vi "SwerveDriveRotate.vi"(0 "Strafe Joystick Axes":cluster{"X":dbl, "Y":dbl}, 1 "Center of Rotation Joystick Axes":cluster{"X":dbl, "Y":dbl}, 3 "Trigger Axes":cluster{"Left":dbl, "Right":dbl}, 4 "Angle (degrees; 0 = right)":dbl, 5 "error in (no error)":errorcluster, 6 "Strafe Multiplier":dbl, 7 "FieldCentric? (T)":bool=TRUE, 8 "Rotation Multiplier":dbl, 10 "Max Wheel Speed":dbl) -> (19 "error out":errorcluster)   [LabVIEW 2014]
uses:
  Robot Global Data.vi
panel:
  in  "Motor Controller":T1(ring)
  out "Waveform Chart":cluster{"FL Speed":dbl, "Encoder Velocity":dbl}(graph)
  in  "set":bool
  in  "D":dbl
  in  "I":dbl
  in  "P":dbl
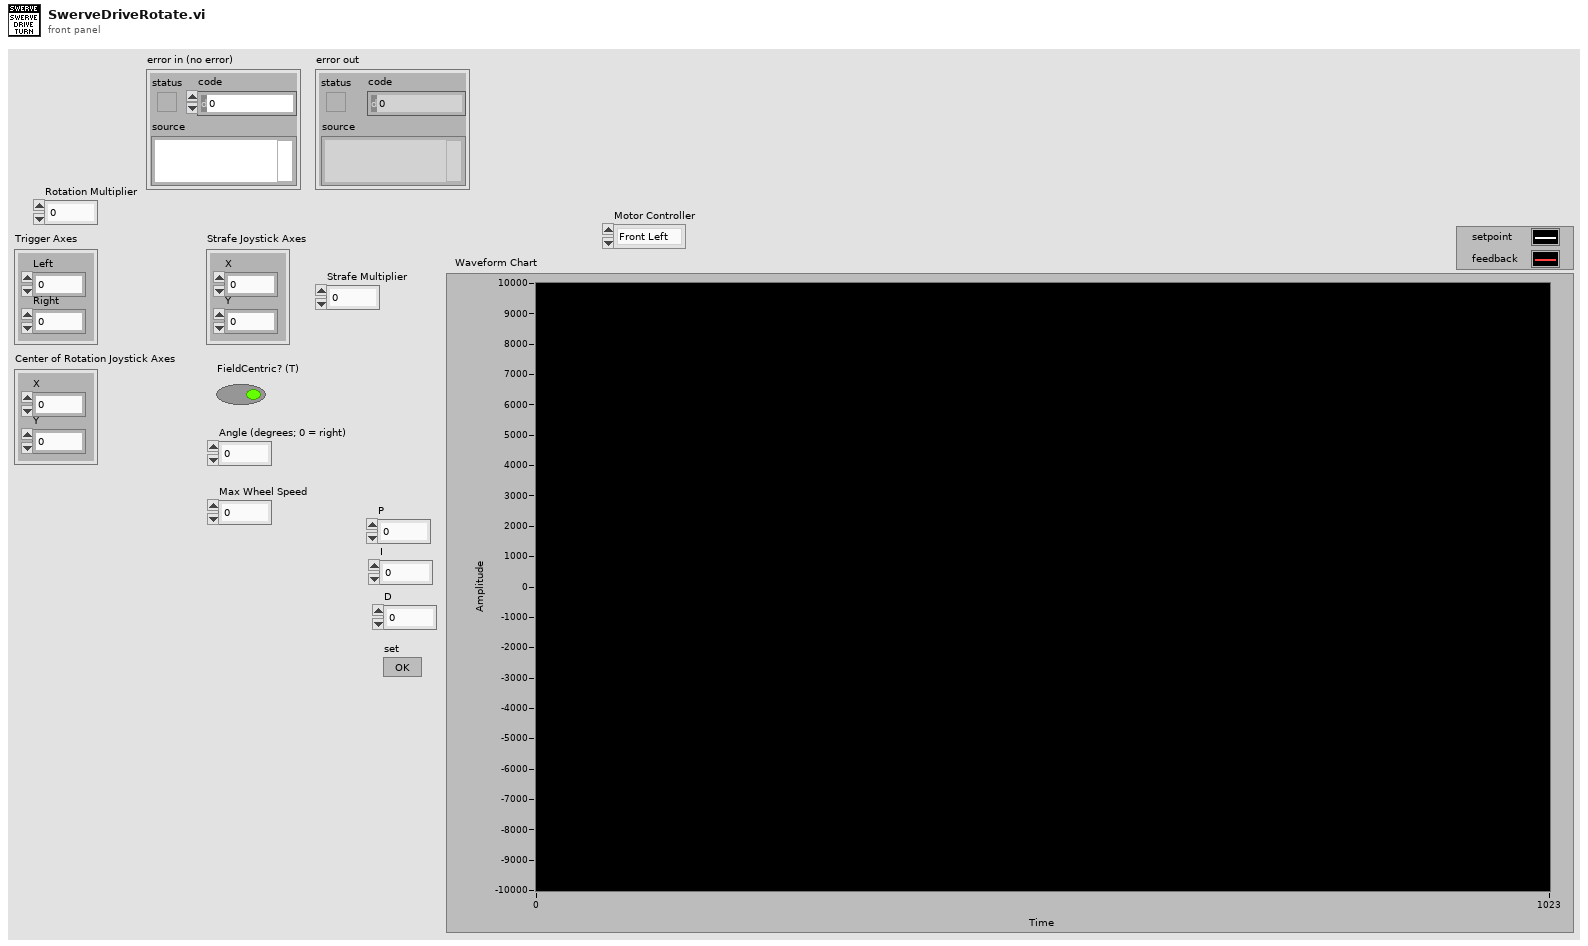
[diagram p1: front panel]
types:
  T1 = enum16{"Front Left", "Front Right", "Rear Left", "Rear Right"}
  T2 = typedef "WPI_MotorControlDeviceRef.ctl" = cluster{"DeviceStatus":errorcluster, "Type":T3, "PWM":cluster{"Controller":T4, "PWM Channel":T5, "DeadBand":T6}, "CAN":cluster{"Device Number":u8, "Control Mode":T7, "Semaphore":T8, "Max Vout":dbl, "TalonSRX Control Mode":T9}, "Invert":bool, "TransformRef":T10, "InvTransformRef":T10}
  T3 = typedef "WPI_MotorControlType.ctl" = enum16{"PWM", "CAN", "CANTalonSRX"}
  T4 = typedef "FPGA_TypedefDigitalModule.ctl" = enum16{"Controller 1"}
  T5 = typedef "FPGA_DIOPWMChannel.ctl" = enum8{"PWM 0", "PWM 1", "PWM 2", "PWM 3", "PWM 4", "PWM 5", "PWM 6", "PWM 7", "PWM 8", "PWM 9", "PWM MXP 0", "PWM MXP 1", "PWM MXP 2", "PWM MXP 3", "PWM MXP 4", "PWM MXP 5", "PWM MXP 6", "PWM MXP 7", "PWM MXP 8", "PWM MXP 9", "Invalid"}
  T6 = typedef "WPI_PWMDeadband.ctl" = cluster{"Name":string, "maxPositivePwm":i32, "minPositivePwm":i32, "centerPwm":i32, "maxNegativePwm":i32, "minNegativePwm":i32, "angularRange":u16}
  T7 = typedef "WPI_CANJaguar_ControlMode.ctl" = enum8{"Percent VBus", "Current", "Speed", "Position", "Voltage"}
  T8 = typedef "Semaphore RefNum" = refnum<k1>
  T9 = typedef "WPI_CANTalonSRX_APIControlMode.ctl" = enum8{"Percent VBus", "Speed", "Position", "Slave", "Unchanged / Invalid"}
  T10 = typedef "WPI_PWMTransform_ConPane.ctl" = refnum<vi>
  T11 = cluster{"FL Steering":T2, "FR Steering":T2, "RL Steering":T2, "RR Steering":T2}
  T12 = cluster{"FL Speed":T2, "FR Speed":T2, "RL Speed":T2, "RR Speed":T2}
  T13 = cluster{"[0]":dbl, "[1]":dbl, "[2]":dbl, "[3]":dbl}
  T14 = typedef "WPI_CANTalonSRX_GlobalStatus.ctl" = cluster{"Applied Throttle":dbl, "Module Enabled":bool, "CAN Error":errorcluster, "Closed Loop Error":dbl, "Forward Limit Switch Closed":bool, "Reverse Limit Switch Closed":bool, "Sensor Position":dbl, "Sensor Velocity":dbl, "Current":dbl, "Sticky Fault - Over Temp":bool, "Sticky Fault - Under Voltage":bool, "Sticky Fault - Forward Limit":bool, "Sticky Fault - Reverse Limit":bool, "Sticky Fault - Forward Soft Limit":bool, "Sticky Fault - Reverse Soft Limit":bool, "Brake is Enabled":bool, "Encoder Position":dbl, "Encoder Velocity":dbl, "Encoder Index Count":dbl, "Encoder A Pin State":bool, "Encoder B Pin State":bool, "Encoder Index Pin State":bool, "Analog In":dbl, "Analog In Velocity":dbl, "Temperature (C)":dbl, "Battery Voltage":dbl}
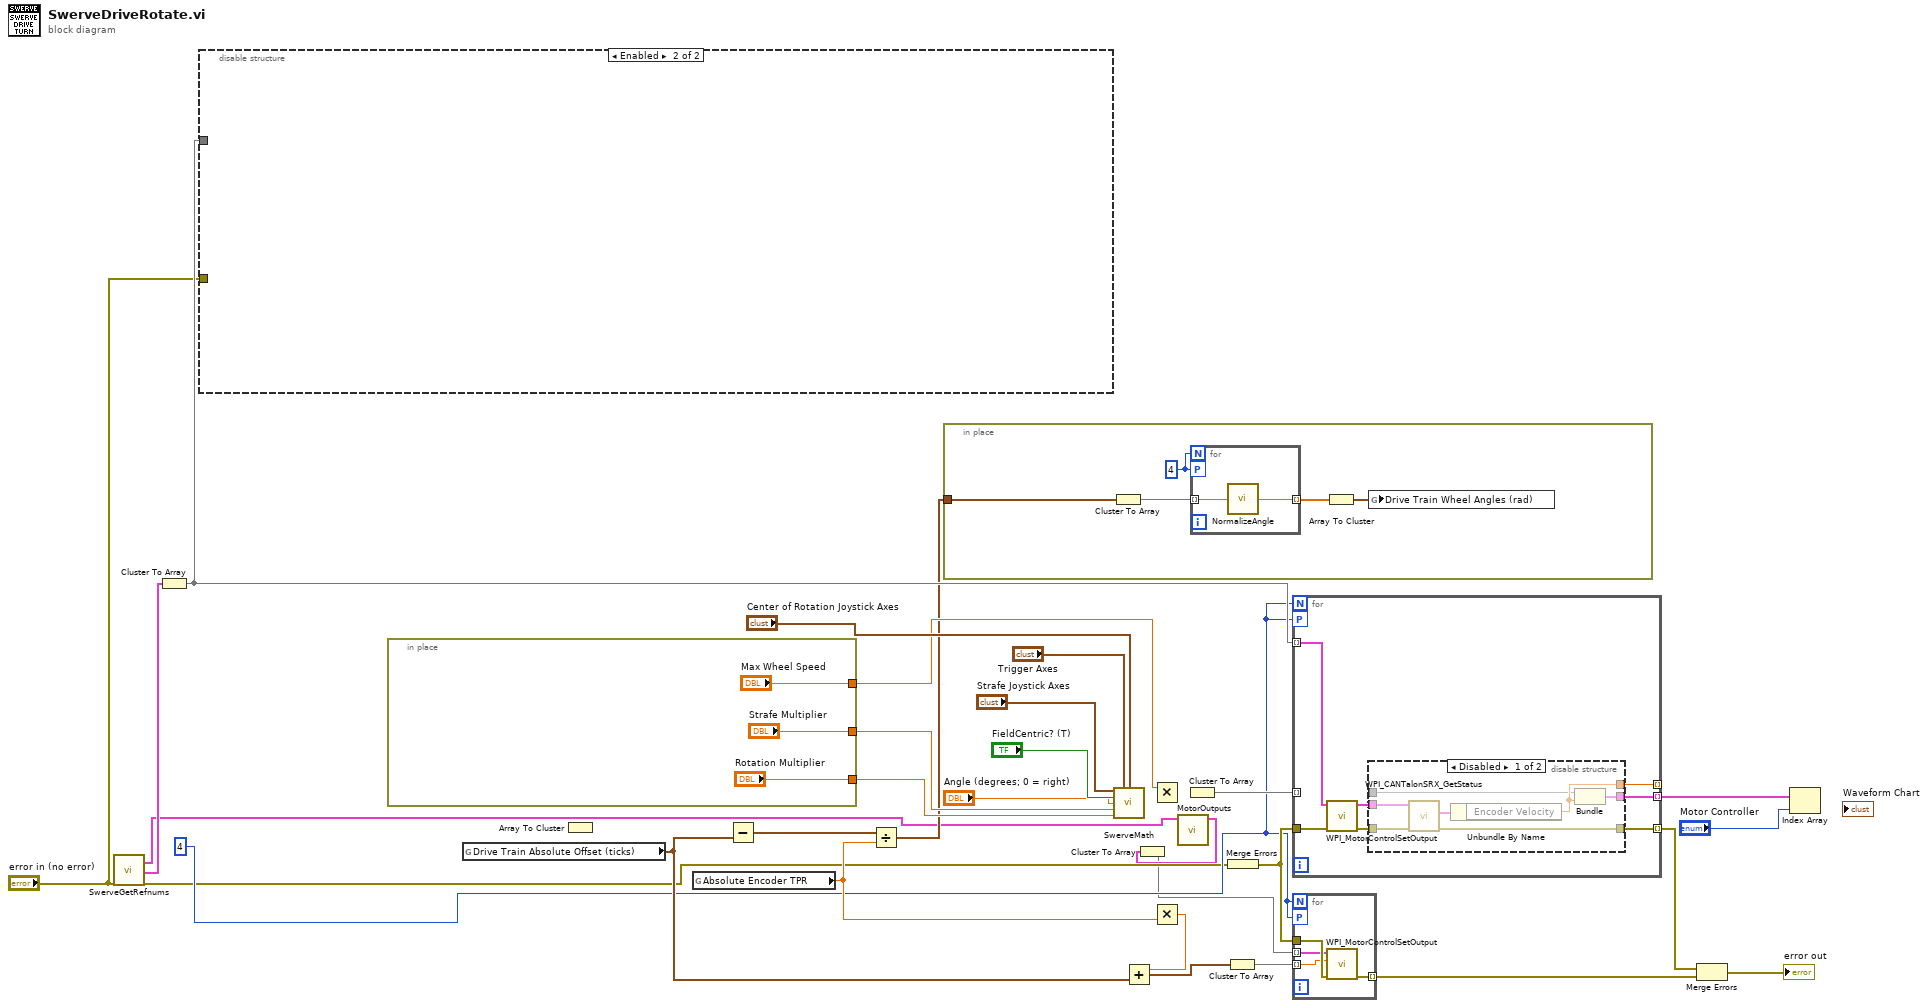
[diagram p0: block diagram]
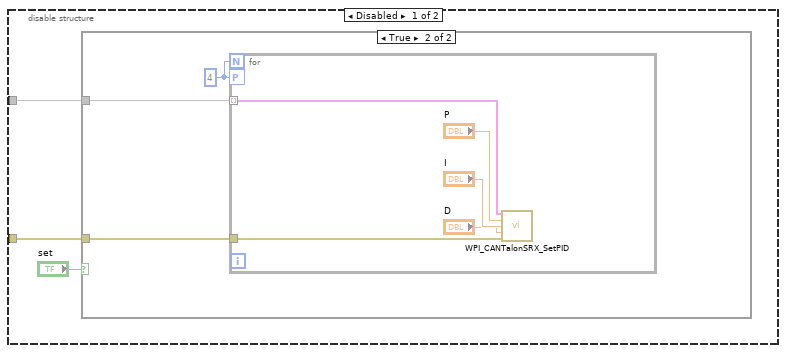
[diagram p2: hidden frame]
diagram:
  w4 = 4
  n1 = call "SwerveGetRefnums.vi"("error in (no error)"="error in (no error)") -> ("Steering"=w5:T11, "Speed"=w23:T12, "error out"=w3:errorcluster)  [unwired: 8 in, 8 out]
  n2 = Cluster To Array(cluster=w23) -> (array=w14:T2[])
  n3 = disable-structure shown="Enabled" {
    disable-tunnel: w14 -> [w33 _]
    disable-tunnel: "error in (no error)" -> [w32 _]
    frame Disabled {
      n4 = case shown="True" "set" {
        tunnel: w33 -> [_ w35]
        tunnel: w32 -> [_ w34]
        frame False {
        }
        frame True {
          w36 = 4
          n5 = for {
            N: w36 -> [_]
            tunnel: w34 -> [w41]
            workers-P: w36 -> [_]
            tunnel: w35 -> [w40] mode=indexing
            n6 = call <vilib>:"WPI_CANTalonSRX_SetPID.vi"("CAN Talon SRX Ref"=w40, "P"="P", "I"="I", "D"="D", "error in (no error)"=w41) -> ()  [unwired: 9 in, 2 out]
          }
        }
      }
    }
    frame Enabled {
    }
  }
  n7 = in-place {
    in-place-border: ["Max Wheel Speed"] -> w8
    in-place-border: ["Rotation Multiplier"] -> w10
    in-place-border: ["Strafe Multiplier"] -> w9
  }
  n8 = global read "Robot Global Data.vi" "Drive Train Absolute Offset (ticks)"() -> (w21:cluster{"FL":dbl, "FR":dbl, "RL":dbl, "RR":dbl})
  n9 = Array To Cluster() -> ()  [unwired: 1 in, 1 out]
  n10 = global read "Robot Global Data.vi" "Absolute Encoder TPR"() -> (w19:dbl)
  n11 = Subtract(y=w21) -> (x-y=w20:cluster{"FL":dbl, "FR":dbl, "RL":dbl, "RR":dbl})  [unwired: 1 in]
  n12 = Divide(x=w20, y=w19) -> (x/y=w6:cluster{"FL":dbl, "FR":dbl, "RL":dbl, "RR":dbl})
  n13 = in-place {
    in-place-border: w6 -> [w46]
    w47 = 4
    n14 = Cluster To Array(cluster=w46) -> (array=w45:dbl[])
    n15 = for {
      N: w47 -> [_]
      tunnel: [w51] -> w49 mode=indexing
      tunnel: w45 -> [w50] mode=indexing
      workers-P: w47 -> [_]
      n16 = call "NormalizeAngle.vi"("angle (rad)"=w50) -> ("angle (between pi and -pi)"=w51:dbl)
    }
    n17 = Array To Cluster(array=w49) -> (cluster=w48:T13)
    n18 = global write "Robot Global Data.vi" "Drive Train Wheel Angles (rad)"(w48) -> ()
  }
  n19 = call "SwerveMath.vi"("Strafe Joystick Axes"="Strafe Joystick Axes", "Trigger Axes"="Trigger Axes", "Center of Rotation Joystick"="Center of Rotation Joystick Axes", "FieldCentric? (T)"="FieldCentric? (T)", "Angle (degrees; 0 = right)"="Angle (degrees; 0 = right)", "Strafe Multiplier"=w9, "Rotation Multiplier"=w10) -> ()  [unwired: 7 in, 2 out]
  n20 = Multiply(x=w8) -> ()  [unwired: 1 in, 1 out]
  n21 = Multiply(y=w19) -> (x*y=w15:dbl)  [unwired: 1 in]
  n22 = Add(x=w15, y=w21) -> (x+y=w16:cluster{"FL":dbl, "FR":dbl, "RL":dbl, "RR":dbl})
  n23 = call "MotorOutputs.vi"("Steering Refnums In"=w5) -> ("Steering Refnums Out"=w2:T11)  [unwired: 7 in, 3 out]
  n24 = Cluster To Array(cluster=w2) -> (array=w1:T2[])
  n25 = Cluster To Array() -> (array=w24:void[])  [unwired: 1 in]
  n26 = Cluster To Array(cluster=w16) -> (array=w22:dbl[])
  n27 = Merge Errors(w3) -> (w7:errorcluster)
  n28 = for {
    N: w4 -> [_]
    tunnel: w7 -> [w58]
    tunnel: [w55] -> w18 mode=indexing
    workers-P: w4 -> [_]
    tunnel: w24 -> [_] mode=indexing
    tunnel: w14 -> [w57] mode=indexing
    tunnel: [w53] -> _ mode=indexing
    tunnel: [w52] -> w12 mode=indexing
    n29 = call <vilib>:"WPI_MotorControlSetOutput.vi"("error in (no error)"=w58, "MotorControlDevRef"=w57) -> ("error out"=w56:errorcluster, "MotorControlDevRef"=w54:T2)  [unwired: 7 in, 1 out]
    n30 = disable-structure shown="Disabled" {
      disable-tunnel: w56 -> [w65 w66]
      disable-tunnel: [w64 w66] -> w55
      disable-tunnel: w54 -> [w63 _]
      disable-tunnel: [w61 _] -> w53
      disable-tunnel: [w59 _] -> w52
      disable-tunnel: _ -> [w60 _]
      frame Disabled {
        n31 = call <vilib>:"WPI_CANTalonSRX_GetStatus.vi"("error in (no error)"=w65, "CAN Talon SRX Ref"=w63) -> ("error out"=w64:errorcluster, "Talon SRX Status"=w62:T14)  [unwired: 7 in, 1 out]
        n32 = Unbundle By Name(w62) -> ("Encoder Velocity"=w61:dbl)
        n33 = Bundle(w60, "Encoder Velocity"=w61) -> (w59:cluster{void, "Encoder Velocity":dbl})  [unwired: 1 in]
      }
      frame Enabled {
      }
    }
  }
  n34 = for {
    N: w4 -> [_]
    tunnel: w7 -> [w70]
    tunnel: [w69] -> w17 mode=indexing
    workers-P: w4 -> [_]
    tunnel: w22 -> [w68] mode=indexing
    tunnel: w1 -> [w67] mode=indexing
    n35 = call <vilib>:"WPI_MotorControlSetOutput.vi"("error in (no error)"=w70, "Output"=w68, "MotorControlDevRef"=w67) -> ("error out"=w69:errorcluster)  [unwired: 6 in, 2 out]
  }
  n36 = Merge Errors(w18, w17) -> (→"error out":errorcluster)
  n37 = Index Array(array=w12, index="Motor Controller") -> ()  [unwired: 1 out]
